vi "stop tasks.vi"(8 "error in (no error)":errorcluster, 11 "Waveform in":refnum<class "Waveform.lvclass">) -> (0 "error out":errorcluster, 3 "Waveform out":refnum<class "Waveform.lvclass">)   [LabVIEW 2012, in "Waveform.lvclass"]
uses:
  Waveform.lvclass
  Waveform.lvclass/Waveform.ctl
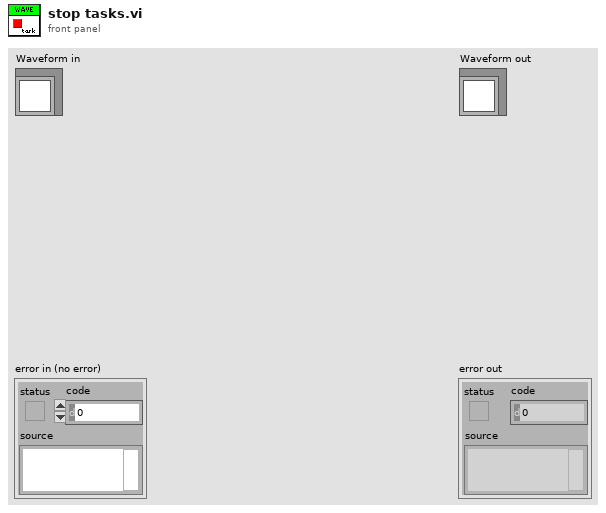
[diagram p1: front panel]
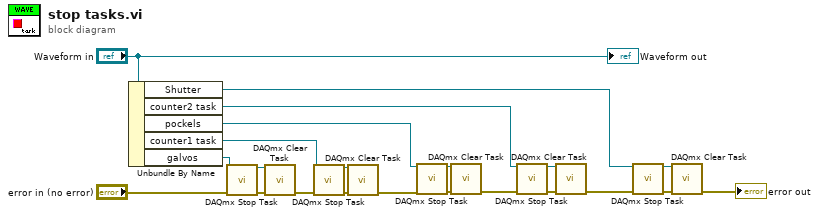
[diagram p0: block diagram]
diagram:
  n1 = Unbundle By Name("Waveform in") -> ("Shutter"=w2:refnum<k21>, "counter2 task"=w7:refnum<k21>, "pockels"=w11:refnum<k21>, "counter1 task"=w15:refnum<k21>, "galvos"=w16:refnum<k21>)
  n2 = call <vilib>:"DAQmx Stop Task.vi"("task/channels in"=w16, "error in"="error in (no error)") -> ("task out"=w18:refnum<k21>, "error out"=w19:errorcluster)  [unwired: 12 in]
  n3 = call <vilib>:"DAQmx Clear Task.vi"("task in"=w18, "error in"=w19) -> ("error out"=w6:errorcluster)  [unwired: 13 in]
  n4 = call <vilib>:"DAQmx Stop Task.vi"("task/channels in"=w15, "error in"=w6) -> ("task out"=w17:refnum<k21>, "error out"=w20:errorcluster)  [unwired: 12 in]
  n5 = call <vilib>:"DAQmx Clear Task.vi"("task in"=w17, "error in"=w20) -> ("error out"=w13:errorcluster)  [unwired: 13 in]
  n6 = call <vilib>:"DAQmx Stop Task.vi"("task/channels in"=w11, "error in"=w13) -> ("task out"=w14:refnum<k21>, "error out"=w12:errorcluster)  [unwired: 12 in]
  n7 = call <vilib>:"DAQmx Clear Task.vi"("task in"=w14, "error in"=w12) -> ("error out"=w9:errorcluster)  [unwired: 13 in]
  n8 = call <vilib>:"DAQmx Stop Task.vi"("task/channels in"=w7, "error in"=w9) -> ("task out"=w10:refnum<k21>, "error out"=w8:errorcluster)  [unwired: 12 in]
  n9 = call <vilib>:"DAQmx Clear Task.vi"("task in"=w10, "error in"=w8) -> ("error out"=w4:errorcluster)  [unwired: 13 in]
  n10 = call <vilib>:"DAQmx Stop Task.vi"("task/channels in"=w2, "error in"=w4) -> ("task out"=w1:refnum<k21>, "error out"=w5:errorcluster)  [unwired: 12 in]
  n11 = call <vilib>:"DAQmx Clear Task.vi"("task in"=w1, "error in"=w5) -> ("error out"=→"error out":errorcluster)  [unwired: 13 in]
  "Waveform out" <- "Waveform in"
